vi "DCC_Get_Init_Status.vi"(8 "Error In":errorcluster, 9 "Ini Status":i16, 10 "ModuleNo":i16, 11 "DLL Path":path) -> (0 "Error Out":errorcluster, 1 "Ini Status":i16, 2 "ModuleNo":i16, 3 "DLL Path":path)   [LabVIEW 2017]
doc: "This procedure loads the ini status variable with the initialisation result code set by the function \"DCC_init Function\" specified by \"Module No.\".\n\nAugust 2018\nFrank Quadt\ninfo@becker-hickl.com"
panel:
  # "(c) 2021 Becker & Hickl GmbH\n     All Rights Reserved."
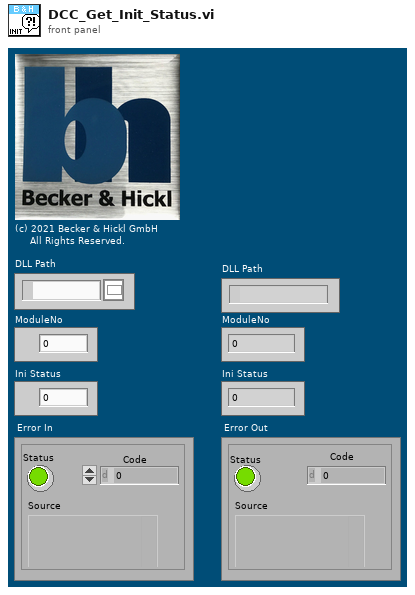
[diagram p1: front panel]
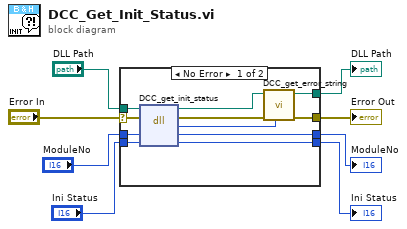
[diagram p0: block diagram]
diagram:
  n1 = case shown="No Error" "Error In" {
    selector: "Error In" -> [w19 w21]
    tunnel: "DLL Path" -> [w18 w23]
    tunnel: [w16 w21] -> w6
    tunnel: [w13 w22] -> w5
    tunnel: "ModuleNo" -> [w12 w22]
    tunnel: [w11 w20] -> w3
    tunnel: "Ini Status" -> [w10 w20]
    tunnel: [w9 w23] -> w1
    frame No Error {
      n2 = dll-call lib="\\\\bh-fs1\\Archiv/FQ/DCC DLL v.2.4/dcc64.dll" fn="DCC_get_init_status"(path in=w18, error in=w19, "ModuleNo"=w12, "IniStatus"=w10) -> (path out=w17:path, error out=w14:errorcluster, "return type"=w15:i16, "ModuleNo"=w13:i16, "IniStatus"=w11:i16)  [unwired: 1 in]
      n3 = call "DCC_get_error_string.vi"("Error ID"=w15, "Error In"=w14, "DLL Path"=w17) -> ("Error Out"=w16:errorcluster, "DLL Path"=w9:path)  [unwired: 6 in, 1 out]
    }
    frame Error {
    }
  }
  "Error Out" <- w6
  "DLL Path" <- w1
  "ModuleNo" <- w5
  "Ini Status" <- w3
